vi "Serial Transfer Simulation.vi"() -> ()   [LabVIEW 2013]
uses:
  <vilib>/rvi/DesktopExecutionNode/Execution/niFpgaDEN_Execute.vi
  <vilib>/rvi/DesktopExecutionNode/DesktopExecutionNode.xnode
  Source/I2S-TDM.lvlib
panel:
  in  "pause":bool
  in  "24-bit data":bool[](array[boolean])=[TRUE, FALSE, FALSE, FALSE, FALSE, FALSE, FALSE, FALSE, FALSE, FALSE, FALSE, FALSE, FALSE, FALSE, FALSE, FALSE, FALSE, FALSE, FALSE, FALSE, FALSE, FALSE, FALSE, TRUE]
  in  "History Size":i32=100
  in  "Reset?":bool
  in  "wait":u32=50
  out "Digital Waveform Graph":digitalwaveform(graph)
  in  "input valid":bool
  in  "transfer length":u8=32
  in  "stop":bool
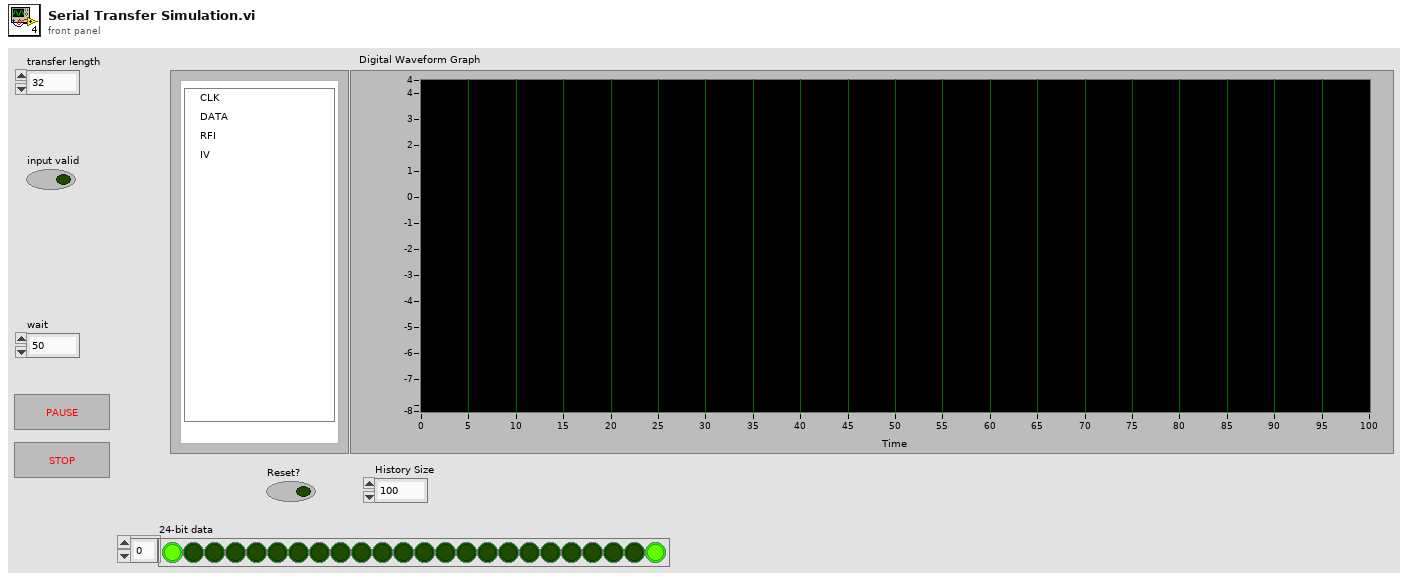
[diagram p1: front panel]
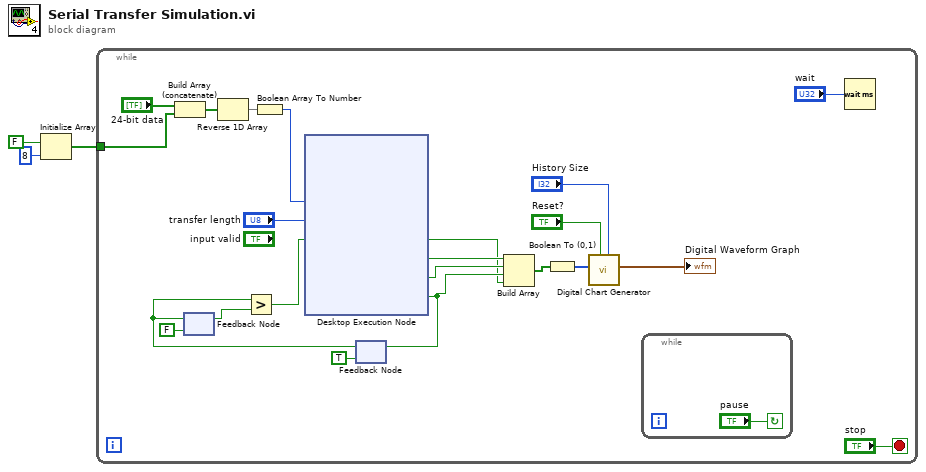
[diagram p0: block diagram]
diagram:
  n1 = Initialize Array(FALSE, 8 ("dimension size")) -> (w1:bool[])
  n2 = while {
    tunnel: w1 -> [w18]
    stop <- "stop" stop-if-true
    n3 = Build Array (concatenate)("24-bit data", w18) -> (w17:bool[])
    n4 = feedback #1(FALSE ("ready for input")) -> (w5:bool)
    n5 = Reverse 1D Array(array=w17) -> (reversed array=w16:bool[])
    n6 = Boolean Array To Number(Boolean array=w16) -> (number=w8:u32)
    n7 = feedback #2(TRUE ("ready for input")) -> (w7:bool)
    n8 = feedback-in #1(w7) -> ()
    n9 = Greater?(x=w7, y=w5) -> (0:w4:bool)
    n10 = xnode "Desktop Execution Node"("sample"=w8, "transfer length"="transfer length", "input valid"=w4) -> ("input valid"=w9:bool, "clk"=w14:bool, "sdata"=w13:bool, "ready for input"=w12:bool)  [unwired: 1 in, 1 out]
    n11 = feedback-in #2(w12) -> ()
    n12 = Build Array(w14, w13, w12, w9) -> (w11:bool[])
    n13 = Boolean To (0,1)(Boolean=w11) -> (0, 1=w10:i16[])
    n14 = call "Digital Chart Generator.vi"("History Size"="History Size", "Reset?"="Reset?", "Input"=w10) -> ("Digital Data"=→"Digital Waveform Graph":digitalwaveform)  [unwired: 8 in]
    n15 = while {
      stop <- "pause" continue-if-true
    }
    n16 = Wait (ms)(milliseconds to wait="wait") -> ()  [unwired: 1 out]
  }
